vi "WPI_MotorControlDisable.vi"(8 "error in (no error)":errorcluster, 11 "MotorControlDevRef":T1={"DeviceStatus"={"status"=FALSE, "code"=0, "source"=""}, "Type"=enum."PWM", "PWM"={"PWM Channel"=enum."Invalid", "DeadBand"={"Name"="", "maxPositivePwm"=0, "minPositivePwm"=0, "centerPwm"=0, "maxNegativePwm"=0, "minNegativePwm"=0, "angularRange"=0}}, "CAN"={"Device Number"=0, "SetOutput VI Ref"=variant(refnum<vi> refnum), "GetOutput VI Ref"=variant(refnum<vi> refnum), "Enable VI Ref"=variant(refnum<vi> refnum), "Disable VI Ref"=variant(refnum<vi> refnum), "Data"=variant}, "Invert"=FALSE, "DIO PWM"={"PWM \"Enable\" Channel"=enum."Invalid", "DIOChannel"=enum."Invalid", "PWM Rate"=0.0}}) -> (0 "error out":errorcluster, 3 "MotorControlDevRef":T1={"DeviceStatus"={"status"=FALSE, "code"=0, "source"=""}, "Type"=enum."PWM", "PWM"={"PWM Channel"=enum."Invalid", "DeadBand"={"Name"="", "maxPositivePwm"=0, "minPositivePwm"=0, "centerPwm"=0, "maxNegativePwm"=0, "minNegativePwm"=0, "angularRange"=0}}, "CAN"={"Device Number"=0, "SetOutput VI Ref"=variant(refnum<vi> refnum), "GetOutput VI Ref"=variant(refnum<vi> refnum), "Enable VI Ref"=variant(refnum<vi> refnum), "Disable VI Ref"=variant(refnum<vi> refnum), "Data"=variant}, "Invert"=FALSE, "DIO PWM"={"PWM \"Enable\" Channel"=enum."Invalid", "DIOChannel"=enum."Invalid", "PWM Rate"=0.0}})   [LabVIEW 2025]
doc: "When the motor controller is connected via PWM, this VI will disable the PWM output on that channel. This is the same behavior that occurs with all PWM outputs in the event of a watchdog error. To resume output, simply call <B>SetOutput</B> again to set a new output VBus percentage.\n\nWhen the motor controller is connected via CAN, this VI will send a message to set output voltage to 0V and stop any running closed-loop controller on the motor controller. After calling this, you must call <B>Enable</B> to resume output and any closed-loop controller.\n\nThis software is licensed. Open the labview\\readme\\WPI Robotics Library Open Source License.txt file for more information."
uses:
  <vilib>/Rock Robotics/WPI/MotorControl/WPI_MotorControlDeviceRef.ctl
  <vilib>/Rock Robotics/WPI/MotorControl/WPI_MotorControlType.ctl
  <vilib>/Rock Robotics/SystemInterfaces/DIO/FPGA_DIOPWMChannel.ctl
  <vilib>/Rock Robotics/WPI/PWM/WPI_PWMDeadband.ctl
  <vilib>/Rock Robotics/SystemInterfaces/DIO/FPGA_DIOChannel.ctl
  <vilib>/Rock Robotics/WPI/PWM/WPI_PWMChannelCacheOp.ctl
  <vilib>/Rock Robotics/WPI/PWM/WPI_PWMSafetyCheck.vi
  <instrlib>/DC Motor Controller/HAIOL/DC Motor Controller.lvclass
  <vilib>/Rock Robotics/WPI/MotorControl/WPI_MotorControlDisableRefType.ctl
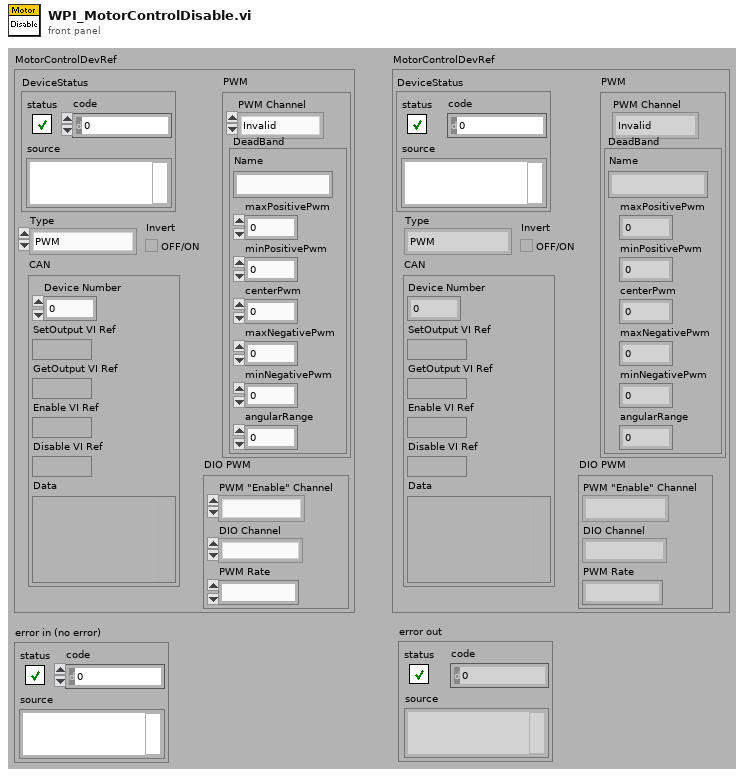
[diagram p1: front panel]
types:
  T1 = typedef "WPI_MotorControlDeviceRef.ctl" = cluster{"DeviceStatus":errorcluster, "Type":T2, "PWM":cluster{"PWM Channel":T3, "DeadBand":T4}, "CAN":cluster{"Device Number":u8, "SetOutput VI Ref":variant, "GetOutput VI Ref":variant, "Enable VI Ref":variant, "Disable VI Ref":variant, "Data":variant}, "Invert":bool, "DIO PWM":cluster{"PWM \"Enable\" Channel":T3, "DIOChannel":T5, "PWM Rate":dbl}}
  T2 = typedef "WPI_MotorControlType.ctl" = enum16{"PWM", "CAN", "DIO PWM"}
  T3 = typedef "FPGA_DIOPWMChannel.ctl" = enum8{"PWM 0", "PWM 1", "PWM 2", "PWM 3", "PWM 4", "PWM 5", "PWM 6", "PWM 7", "PWM 8", "PWM 9", "PWM MXP 0", "PWM MXP 1", "PWM MXP 2", "PWM MXP 3", "PWM MXP 4", "PWM MXP 5", "PWM MXP 6", "PWM MXP 7", "PWM MXP 8", "PWM MXP 9", "Invalid"}
  T4 = typedef "WPI_PWMDeadband.ctl" = cluster{"Name":string, "maxPositivePwm":i32, "minPositivePwm":i32, "centerPwm":i32, "maxNegativePwm":i32, "minNegativePwm":i32, "angularRange":u16}
  T5 = typedef "FPGA_DIOChannel.ctl" = enum8{"DIO 0", "DIO 1", "DIO 2", "DIO 3", "DIO 4", "DIO 5", "DIO 6", "DIO 7", "DIO 8", "DIO 9", "DIO MXP 0", "DIO MXP 1", "DIO MXP 2", "DIO MXP 3", "DIO MXP 4", "DIO MXP 5", "DIO MXP 6", "DIO MXP 7", "DIO MXP 8", "DIO MXP 9", "DIO MXP 10", "DIO MXP 11", "DIO MXP 12", "DIO MXP 13", "DIO MXP 14", "DIO MXP 15", "SPI Port CS1", "SPI Port CS2", "SPI Port CS3", "SPI Port MISO", "SPI Port MOSI", "Invalid"}
  T6 = typedef "WPI_MotorControlDisableRefType.ctl" = refnum<vi>
  T7 = typedef "WPI_PWMChannelCacheOp.ctl" = enum16{"Acquire", "Release", "Status"}
  T8 = typedef "WPI_PWMDeviceRef.ctl" = cluster{"DeviceStatus":errorcluster, "PWM Channel":T3}
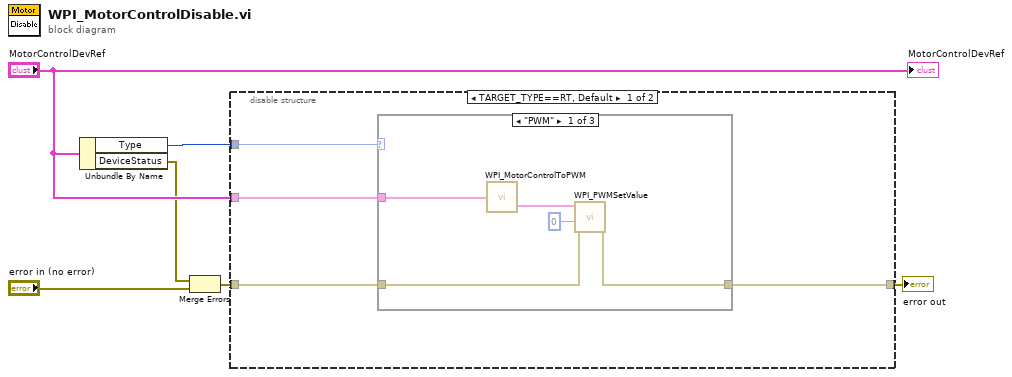
[diagram p0: block diagram]
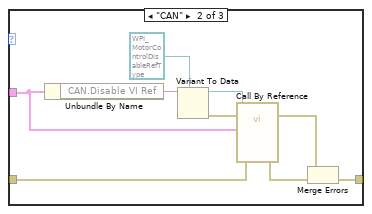
[diagram p2: hidden frame]
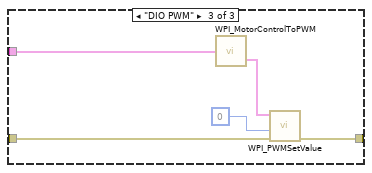
[diagram p3: hidden frame]
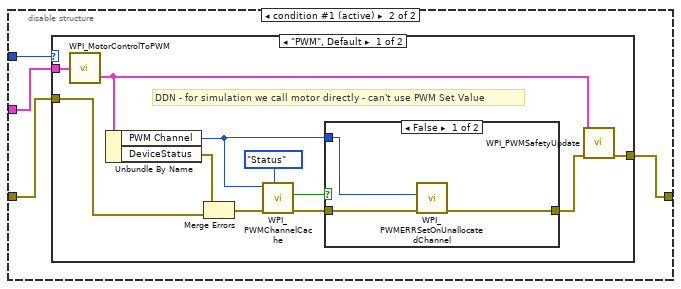
[diagram p4: hidden frame]
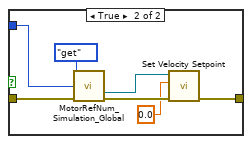
[diagram p5: hidden frame]
diagram:
  n1 = Unbundle By Name("MotorControlDevRef") -> ("Type"=w4:T2, "DeviceStatus"=w3:errorcluster)
  n2 = Merge Errors(w3, "error in (no error)") -> (w1:errorcluster)
  n3 = disable-structure shown="TARGET_TYPE==RT, Default" {
    disable-tunnel: [w10 w33] -> w6
    disable-tunnel: "MotorControlDevRef" -> [w9 w30]
    disable-tunnel: w4 -> [w8 w31]
    disable-tunnel: w1 -> [w7 w32]
    frame condition #0 {
      n4 = case shown="\"PWM\"" w8 {
        tunnel: w7 -> [w12 w24 w29]
        tunnel: [w11 w18 w28] -> w10
        tunnel: w9 -> [w14 w23 w26]
        frame "PWM" {
          n5 = call <vilib>:"WPI_MotorControlToPWM.vi"("MotorControlDeviceRef"=w14) -> ("PWMDeviceRef"=w15:T8)  [unwired: 1 out]
          n6 = call <vilib>:"WPI_PWMSetValue.vi"("error in (no error)"=w12, "Value"=u16 0, "PWMDeviceRef"=w15) -> ("error out"=w11:errorcluster)  [unwired: 1 in, 7 out]
        }
        frame "CAN" {
          n7 = Unbundle By Name(w23) -> ("CAN.Disable VI Ref"=w22:variant)
          n8 = Variant To Data(type=T6 refnum ("MotorControlSetOutput"), Variant=w22) -> (data=w21:T6, error out=w20:errorcluster)  [unwired: 1 in]
          n9 = call-by-ref "?"(reference=w21, error in=w20, 8:"error in (no error)"=w24, "MotorControlDevRef"=w23) -> (error out=w17:errorcluster, 0:"error out"=w19:errorcluster)  [unwired: 8 in, 2 out]
          n10 = Merge Errors(w17, w19) -> (w18:errorcluster)
        }
        frame "DIO PWM" {
          n11 = call <vilib>:"WPI_MotorControlToPWM.vi"("MotorControlDeviceRef"=w26) -> ("PWMDeviceRef"=w25:T8)  [unwired: 1 out]
          n12 = call <vilib>:"WPI_PWMSetValue.vi"("error in (no error)"=w29, "Value"=u16 0, "PWMDeviceRef"=w25) -> ("error out"=w28:errorcluster)  [unwired: 7 in, 1 out]
        }
      }
    }
    frame condition #1 (active) {
      n13 = case shown="\"PWM\", Default" w31 {
        tunnel: w32 -> [w36 w55]
        tunnel: [w35 w55] -> w33
        tunnel: w30 -> [w44 _]
        frame "PWM", Default {
          # "DDN - for simulation we call motor directly - can't use PWM Set Value"
          n14 = call <vilib>:"WPI_MotorControlToPWM.vi"("MotorControlDeviceRef"=w44) -> ("PWMDeviceRef"=w34:T8)  [unwired: 1 out]
          n15 = Unbundle By Name(w34) -> ("PWM Channel"=w40:T3, "DeviceStatus"=w38:errorcluster)
          n16 = Merge Errors(w38, w36) -> (w39:errorcluster)
          n17 = call <vilib>:"WPI_PWMChannelCache.vi"("Operation"=WPI_PWMChannelCacheOp."Status", "error in (no error)"=w39, "PWMChannel"=w40) -> ("error out"=w42:errorcluster, "Allocated?"=w41:bool)  [unwired: 2 in, 5 out]
          n18 = case shown="False" w41 {
            tunnel: w42 -> [w47 w53]
            tunnel: [w46 w49] -> w43
            tunnel: w40 -> [w45 w51]
            frame False {
              n19 = call <vilib>:"WPI_PWMERRSetOnUnallocatedChannel.vi"("error in (no error)"=w47, "PWM Channel"=w45) -> ("error out"=w46:errorcluster)  [unwired: 9 in]
            }
            frame True {
              n20 = call <vilib>:"MotorRefNum_Simulation_Global.vi"("menu"=enum16{"set", "get", "delete"}."get", "PWM Channel"=w51, "error in (no error)"=w53) -> ("DC Motor Controller Get"=w50:refnum<class "DC Motor Controller.lvclass">, "error out"=w52:errorcluster)  [unwired: 11 in]
              n21 = call-dynamic "Set Velocity Setpoint.vi"("error in (no error)"=w52, "CCW Velocity (0 rad/s)"=0.0, "DC Motor Controller in"=w50) -> ("error out"=w49:errorcluster)  [unwired: 7 in, 1 out]
            }
          }
          n22 = call <vilib>:"WPI_PWMSafetyUpdate.vi"("error in (no error)"=w43, "PWMDeviceRef"=w34) -> ("error out"=w35:errorcluster)  [unwired: 9 out]
        }
        frame "CAN" {
        }
      }
    }
  }
  "error out" <- w6
  "MotorControlDevRef" <- "MotorControlDevRef"
